vi "handleIncomingMessages_old.vi"(8 "error in (no error)":errorcluster, 11 "DataListenerThisComponent in":refnum<class "DataListenerThisComponent.lvclass">) -> (0 "error out":errorcluster, 3 "DataListenerThisComponent out":refnum<class "DataListenerThisComponent.lvclass">)   [LabVIEW 2015]
uses:
  UserEventsThisComponent/UserEventsThisComponent.lvclass
  ComponentTemplateCore/ComponentModel/ComponentModel/UserEvents/UserEvents.lvclass
  Typedefs/CommandValue.ctl
  Typedefs/EXATypedefs.lvlib
  ICommandFactory/ICommandFactory.lvclass
  ComponentTemplateCore/ComponentModel/ComponentModel/DataListener/DataListener.lvclass
  DataListenerThisComponent.lvclass
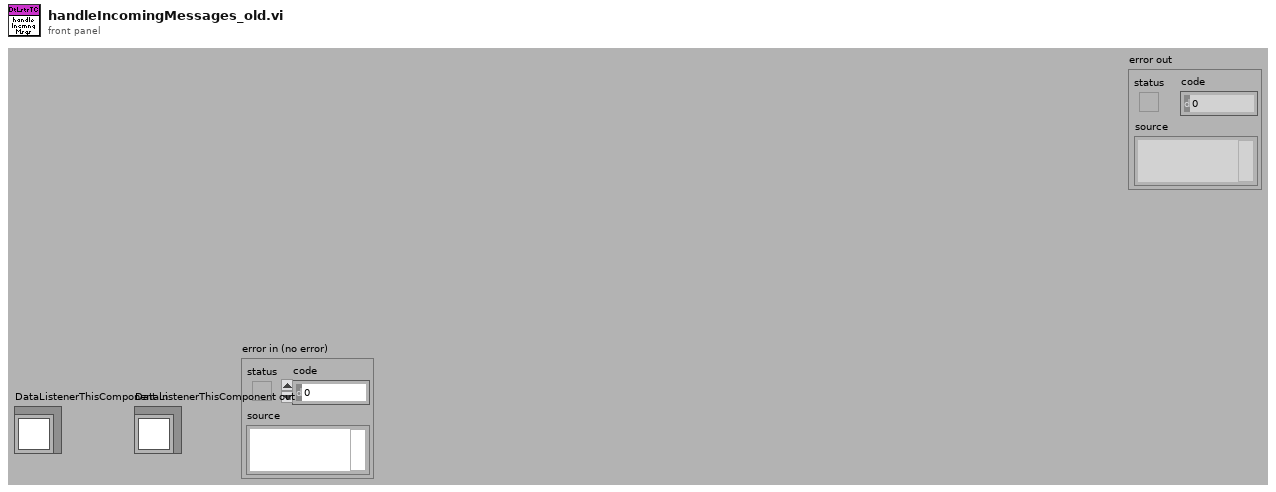
[diagram p1: front panel]
types:
  T1 = typedef "EXATypedefs.lvlib/CommandEvents.ctl" = cluster{"command":refnum<user-event>}
  T2 = typedef "EXATypedefs.lvlib/SubDataEvents.ctl" = cluster{"ClearError":refnum<user-event>, "Disable":refnum<user-event>, "Enable":refnum<user-event>, "Exit":refnum<user-event>, "GoToStandby":refnum<user-event>, "HeartbeatIn":refnum<user-event>, "Start":refnum<user-event>}
  T3 = typedef "EXATypedefs.lvlib/CommandValue.ctl" = enum16{"ClearError", "Disable", "Enable", "Exit", "GoToStandby", "OnHeartbeat", "OnIncomingMessagingError", "OnInterrupt", "Start"}
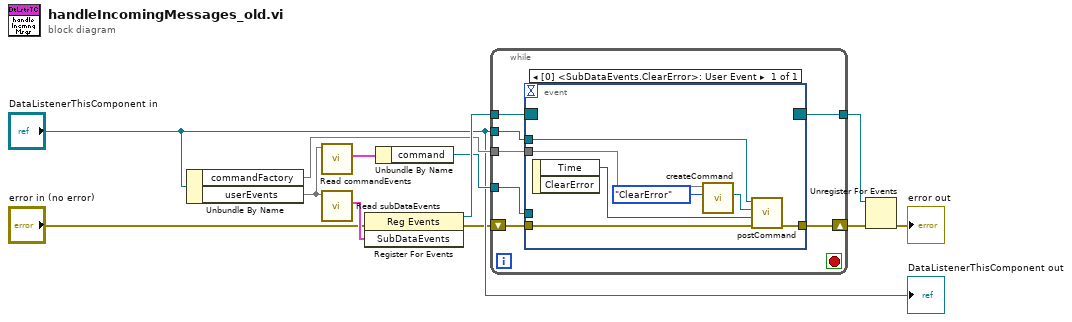
[diagram p0: block diagram]
diagram:
  n1 = Unbundle By Name("DataListenerThisComponent in") -> ("commandFactory"=w8, "userEvents"=w12)
  n2 = call "Read commandEvents.vi"("UserEvents in"=w12) -> ("CommandEvents"=w7:T1)  [unwired: 9 in, 1 out]
  n3 = call "Read subDataEvents.vi"("UserEventsThisComponent in"=w12) -> ("SubDataEvents"=w11:T2)  [unwired: 9 in, 1 out]
  n4 = register-events(error in="error in (no error)", w11) -> (reference out=w10:refnum<event-registration>, error out=w4:errorcluster)  [unwired: 1 in]
  n5 = Unbundle By Name(w7) -> ("command"=w6:refnum<user-event>)
  n6 = while {
    tunnel: w10 -> [w19]
    tunnel: [w18] -> w9
    tunnel: w8 -> [w17]
    tunnel: w6 -> [w16]
    tunnel: "DataListenerThisComponent in" -> [w15]
    shift-right: [w13] -> w2
    shift-left: w4 -> [w14]
    stop <- _ stop-if-true
    n7 = event shown="[0] <SubDataEvents.ClearError>: User Event" {
      selector: w19 -> [_]
      dyn-events: [_] -> w18
      timeout: _ -> [_]
      tunnel: w17 -> [w25]
      tunnel: w16 -> [_]
      tunnel: w15 -> [w23]
      tunnel: w14 -> [w21]
      tunnel: [w20] -> w13
      event User Event {
        n8 = event-data() -> ("Time"=w22:u32)  [unwired: 1 in, 1 out]
        n9 = call-dynamic "createCommand.vi"("commandValue"=CommandValue."ClearError", "ICommandFactory in"=w25) -> ("command"=w24:refnum<class "Command.lvclass">)  [unwired: 7 in, 2 out]
        n10 = call "postCommand.vi"("error in (no error)"=w21, "Time"=w22, "command"=w24, "DataListener in"=w23) -> ("error out"=w20:errorcluster)  [unwired: 6 in, 1 out]
      }
    }
  }
  n11 = Unregister For Events(event registration refnum=w9, error in=w2) -> (error out=→"error out":errorcluster)
  "DataListenerThisComponent out" <- "DataListenerThisComponent in"
